vi "Reproductor.vi"() -> ()   [LabVIEW 2016]
uses:
  <vilib>/sound2/lvsound2.llb/Sound Data Format.ctl
  <vilib>/sound2/lvsound2.llb/Sound File Position.ctl
  <vilib>/sound2/lvsound2.llb/Sampling Mode.ctl
  <vilib>/Analysis/baseanly.llb/Mean (DBL).vi
  <vilib>/sound2/lvsound2.llb/Sound File Read Open.vi
  <vilib>/sound2/lvsound2.llb/Sound File Info (refnum).vi
  <vilib>/sound2/lvsound2.llb/Sound File Read (DBL).vi
  <vilib>/measure/matone.llb/Extract Single Tone Information N Chan.vi
  <vilib>/measure/maspectr.llb/FFT Spectrum (Mag-Phase) for N Chan.vi
  <vilib>/sound2/lvsound2.llb/Sound Output Write (DBL).vi
  <vilib>/measure/NI_MAPro.lvlib
  <vilib>/Analysis/NI_AALBase.lvlib
panel:
  in  "Skip Forward Button":bool
  in  "Seek Forward Button":bool
  in  "Pause Button":bool
  in  "Play Button":bool
  in  "Seek Back Button":bool
  in  "Skip Back Button":bool
  in  "posicion":dbl(slide) scale=0.0..10.0
  out "Color Box":u32(colorbox)
  out "Waveform Chart":cluster{"mean":dbl, "detected frequency":dbl}(graph)
  out "Waveform Graph 2":cluster{"f0":dbl, "df":dbl, "magnitude":dbl[]}[](graph)
  in  "stop":bool
  out "Waveform Graph":waveform(dbl)[](graph)
  out "sound format":T1={"sample rate (S/s)"=22050.0, "number of channels"=2, "bits per sample"=16}
  out "total number of samples/ch":u32
  in  "path":path=path "C:/Users/jesus/Desktop/Reproductor/Shawn Mendes  Bad Reputation    Traducido al Español.wav"
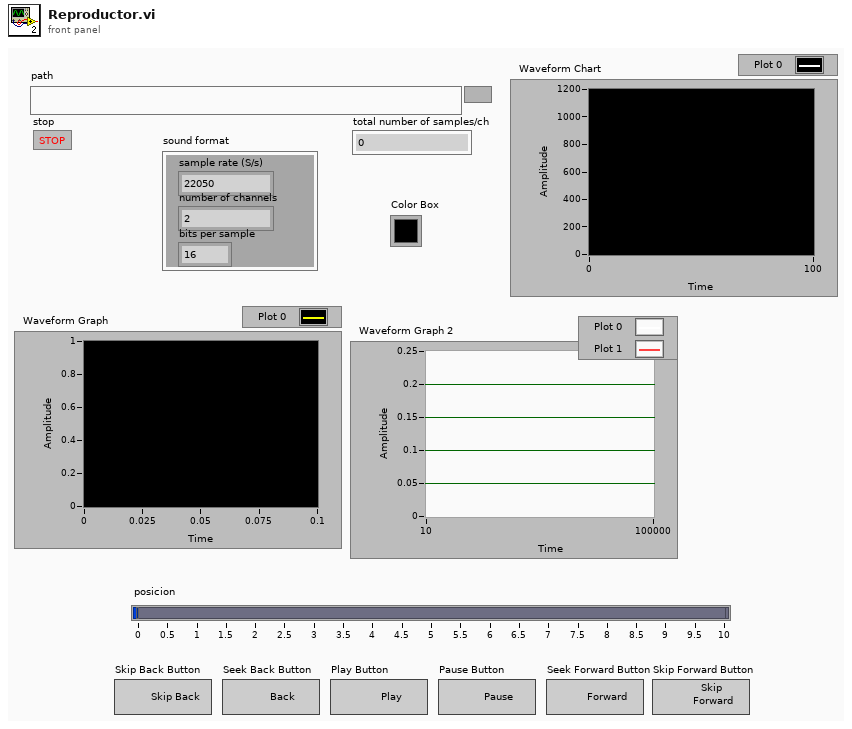
[diagram p1: front panel]
types:
  T1 = typedef "Sound Data Format.ctl" = cluster{"sample rate (S/s)":dbl, "number of channels":i32, "bits per sample":i32}
  T2 = typedef "Sampling Mode.ctl" = i32
  T3 = typedef "Sound File Position.ctl" = u16
  T4 = typedef "Sound File Refnum.ctl" = refnum<file>
  T5 = typedef "Sound Output Task ID.ctl" = u32
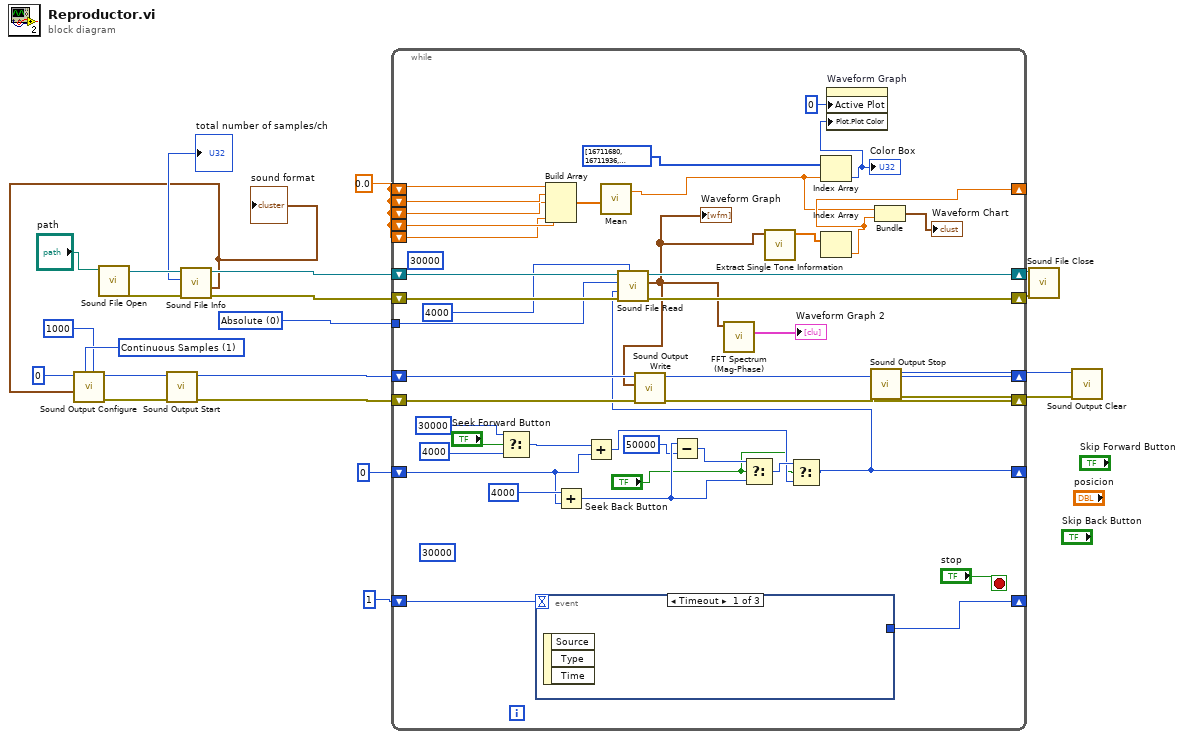
[diagram p0: block diagram]
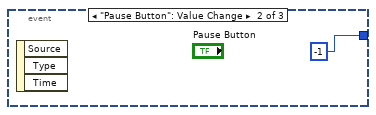
[diagram p2: hidden frame]
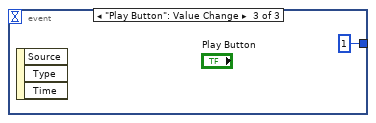
[diagram p3: hidden frame]
diagram:
  w3 = 0.0 ("detected frequency")
  w13 = T2 1 items=["Finite Samples", "Continuous Samples"] ("sample mode")
  w16 = T3 0 items=["Absolute"=0, "Relative"=2] ("position mode")
  n1 = call-poly <vilib>:"Sound File Open.vi"("path"="path") -> ("error out"=w22:errorcluster, "sound file refnum"=w23:T4)  [unwired: 9 in]
  n2 = call-poly <vilib>:"Sound File Info.vi"("error in (no error)"=w22, "sound file refnum"=w23) -> ("error out"=w19:errorcluster, "sound format"=w14:T1, "total number of samples/ch"=→"total number of samples/ch":u32, "sound file refnum out"=w20:T4)  [unwired: 6 in]
  "sound format" <- w14
  n3 = call <vilib>:"Sound Output Configure.vi"("number of samples/ch"=1000, "sample mode"=w13, "sound format"=w14, "device ID"=u32 0) -> ("error out"=w10:errorcluster, "task ID"=w11:T5)  [unwired: 6 in]
  n4 = call <vilib>:"Sound Output Start.vi"("error in (no error)"=w10, "task ID"=w11) -> ("error out"=w8:errorcluster, "task ID out"=w9:T5)  [unwired: 8 in]
  n5 = while {
    tunnel: w16 -> [w61]
    shift-right: [w63] -> w18
    shift-left: w20 -> [w65]
    shift-right: [w62] -> w17
    shift-left: w19 -> [w64]
    shift-right: [w58] -> w7
    shift-left: w9 -> [w60]
    shift-right: [w57] -> w5
    shift-left: w8 -> [w59]
    shift-right: [w46] -> _
    shift-left: w3 -> [w50]
    shift-left: w3 -> [w51]
    shift-left: w3 -> [w49]
    shift-left: w3 -> [w48]
    shift-left: w3 -> [w41]
    shift-right: [w27] -> _
    shift-left: 0 -> [w32]
    shift-right: [w40] -> _
    shift-left: 1 -> [w39]
    stop <- "stop" stop-if-true
    (unwired) 30000 ("number of samples/ch (-1: all)")
    (unwired) 30000 ("number of samples/ch (-1: all)")
    n6 = Select(t=30000 ("number of samples/ch (-1: all)"), s="Seek Forward Button", f=4000) -> (s? t:f=w38:i32)
    n7 = event shown="[0] Timeout" {
      selector: _ -> [_ _ _]
      dyn-events: _ -> [_ _ _]
      timeout: w39 -> [_ _ _]
      tunnel: [_ -1 1] -> w40
      event Timeout {
        n8 = event-data() -> ()  [unwired: 1 in, 3 out]
      }
      event "Pause Button": Value Change {
        n9 = event-data() -> ()  [unwired: 1 in, 3 out]
      }
      event "Play Button": Value Change {
        n10 = event-data() -> ()  [unwired: 1 in, 3 out]
      }
    }
    n11 = Build Array(w50, w51, w49, w48, w41) -> (w47:dbl[])
    n12 = Add(x=4000, y=w32) -> (x+y=w30:i32)
    n13 = Add(x=w38, y=w32) -> (x+y=w26:i32)
    n14 = call-poly <vilib>:"Mean.vi"("X"=w47) -> ("mean"=w45:dbl)  [unwired: 1 out]
    n15 = Subtract(x=w30, y=50000 ("x")) -> (x-y=w31:i32)
    n16 = Select(t=w31, s="Seek Back Button", f=w30) -> (s? t:f=w28:i32)
    n17 = Select(t=w28, s="Seek Back Button", f=w26) -> (s? t:f=w27:i32)
    n18 = call-poly <vilib>:"Sound File Read.vi"("number of samples/ch (-1: all)"=4000, "error in (no error)"=w64, "position offset"=w27, "position mode"=w61, "sound file refnum"=w65) -> ("error out"=w62:errorcluster, "data"=w54:waveform(dbl)[], "sound file refnum out"=w63:T4)  [unwired: 2 in, 2 out]
    "Waveform Graph" <- w54
    n19 = call-poly <vilib>:"Sound Output Write.vi"("error in (no error)"=w59, "data"=w54, "task ID"=w60) -> ("error out"=w57:errorcluster, "task ID out"=w58:T5)  [unwired: 7 in]
    n20 = call-poly <vilib>:"FFT Spectrum (Mag-Phase).vi"("time signals"=w54) -> ("magnitudes"=→"Waveform Graph 2":cluster{"f0":dbl, "df":dbl, "magnitude":dbl[]}[])  [unwired: 6 in, 4 out]
    n21 = call-poly <vilib>:"Extract Single Tone Information.vi"("time signals in"=w54) -> ("detected frequencies"=w53:dbl[])  [unwired: 5 in, 5 out]
    n22 = Index Array(array=u32[] [16711680, 16711936, 16712192, 16712448, 16712704, 16712960, 16713216, 16713472, 16713728, 16713984, 16714240, 16714496, 16714752, 16715008, 16715264, 16715520, 16715776, 16716032, 16716288, 16716544, 16716800, 16717056, 16717312, 16717568, 16717824, 16718080, 16718336, 16718592, 16718848, 16719104, 16719360, 16719616, 16719872, 16720128, 16720384, 16720640, 16720896, 16721152, 16721408, 16721664, 16721920, 16722176, 16722432, 16722688, 16722944, 16723200, 16723456, 16723712, 16723968, 16724224, 16724480, 16724736, 16724992, 16725248, 16725504, 16725760, 16726016, 16726272, 16726528, 16726784, 16727040, 16727296, 16727552, 16727808, 16728064, 16728320, 16728576, 16728832, 16729088, 16729344, 16729600, 16729856, 16730112, 16730368, 16730624, 16730880, 16731136, 16731392, 16731648, 16731904, 16732160, 16732416, 16732672, 16732928, 16733184, 16733440, 16733696, 16733952, 16734208, 16734464, 16734720, 16734976, 16735232, 16735488, 16735744, 16736000, 16736256, 16736512, 16736768, 16737024, 16737280, 16737536, 16737792, 16738048, 16738304, 16738560, 16738816, 16739072, 16739328, 16739584, 16739840, 16740096, 16740352, 16740608, 16740864, 16741120, 16741376, 16741632, 16741888, 16742144, 16742400, 16742656, 16742912, 16743168, 16743424, 16743680, 16743936, 16744192, 16744448, 16744704, 16744960, 16745216, 16745472, 16745728, 16745984, 16746240, 16746496, 16746752, 16747008, 16747264, 16747520, 16747776, 16748032, 16748288, 16748544, 16748800, 16749056, 16749312, 16749568, 16749824, 16750080, 16750336, 16750592, 16750848, 16751104, 16751360, 16751616, 16751872, 16752128, 16752384, 16752640, 16752896, 16753152, 16753408, 16753664, 16753920, 16754176, 16754432, 16754688, 16754944, 16755200, 16755456, 16755712, 16755968, 16756224, 16756480, 16756736, 16756992, 16757248, 16757504, 16757760, 16758016, 16758272, 16758528, 16758784, 16759040, 16759296, 16759552, 16759808, 16760064, 16760320, 16760576, 16760832, 16761088, 16761344, 16761600, 16761856, 16762112, 16762368, 16762624, 16762880, 16763136, 16763392, 16763648, 16763904, 16764160, 16764416, 16764672, 16764928, 16765184, 16765440, 16765696, 16765952, 16766208, 16766464, 16766720, 16766976, 16767232, 16767488, 16767744, 16768000, 16768256, 16768512, 16768768, 16769024, 16769280, 16769536, 16769792, 16770048, 16770304, 16770560, 16770816, 16771072, 16771328, 16771584, 16771840, 16772096, 16772352, 16772608, 16772864, 16773120, 16773376, 16773632, 16773888, 16774144, 16774400, 16774656, 16774912, 16775168, 16775424, 16775680, 16775936, 16776192, 16776448, 16776704, 16776960, 16711424, 16645888, 16580352, 16514816, 16449280, 16383744, 16318208, 16252672, 16187136, 16121600, 16056064, 15990528, 15924992, 15859456, 15793920, 15728384, 15662848, 15597312, 15531776, 15466240, 15400704, 15335168, 15269632, 15204096, 15138560, 15073024, 15007488, 14941952, 14876416, 14810880, 14745344, 14679808, 14614272, 14548736, 14483200, 14417664, 14352128, 14286592, 14221056, 14155520, 14089984, 14024448, 13958912, 13893376, 13827840, 13762304, 13696768, 13631232, 13565696, 13500160, 13434624, 13369088, 13303552, 13238016, 13172480, 13106944, 13041408, 12975872, 12910336, 12844800, 12779264, 12713728, 12648192, 12582656, 12517120, 12451584, 12386048, 12320512, 12254976, 12189440, 12123904, 12058368, 11992832, 11927296, 11861760, 11796224, 11730688, 11665152, 11599616, 11534080, 11468544, 11403008, 11337472, 11271936, 11206400, 11140864, 11075328, 11009792, 10944256, 10878720, 10813184, 10747648, 10682112, 10616576, 10551040, 10485504, 10419968, 10354432, 10288896, 10223360, 10157824, 10092288, 10026752, 9961216, 9895680, 9830144, 9764608, 9699072, 9633536, 9568000, 9502464, 9436928, 9371392, 9305856, 9240320, 9174784, 9109248, 9043712, 8978176, 8912640, 8847104, 8781568, 8716032, 8650496, 8584960, 8519424, 8453888, 8388352, 8322816, 8257280, 8191744, 8126208, 8060672, 7995136, 7929600, 7864064, 7798528, 7732992, 7667456, 7601920, 7536384, 7470848, 7405312, 7339776, 7274240, 7208704, 7143168, 7077632, 7012096, 6946560, 6881024, 6815488, 6749952, 6684416, 6618880, 6553344, 6487808, 6422272, 6356736, 6291200, 6225664, 6160128, 6094592, 6029056, 5963520, 5897984, 5832448, 5766912, 5701376, 5635840, 5570304, 5504768, 5439232, 5373696, 5308160, 5242624, 5177088, 5111552, 5046016, 4980480, 4914944, 4849408, 4783872, 4718336, 4652800, 4587264, 4521728, 4456192, 4390656, 4325120, 4259584, 4194048, 4128512, 4062976, 3997440, 3931904, 3866368, 3800832, 3735296, 3669760, 3604224, 3538688, 3473152, 3407616, 3342080, 3276544, 3211008, 3145472, 3079936, 3014400, 2948864, 2883328, 2817792, 2752256, 2686720, 2621184, 2555648, 2490112, 2424576, 2359040, 2293504, 2227968, 2162432, 2096896, 2031360, 1965824, 1900288, 1834752, 1769216, 1703680, 1638144, 1572608, 1507072, 1441536, 1376000, 1310464, 1244928, 1179392, 1113856, 1048320, 982784, 917248, 851712, 786176, 720640, 655104, 589568, 524032, 458496, 392960, 327424, 261888, 196352, 130816, 65280, 65281, 65282, 65283, 65284, 65285, 65286, 65287, 65288, 65289, 65290, 65291, 65292, 65293, 65294, 65295, 65296, 65297, 65298, 65299, 65300, 65301, 65302, 65303, 65304, 65305, 65306, 65307, 65308, 65309, 65310, 65311, 65312, 65313, 65314, 65315, 65316, 65317, 65318, 65319, 65320, 65321, 65322, 65323, 65324, 65325, 65326, 65327, 65328, 65329, 65330, 65331, 65332, 65333, 65334, 65335, 65336, 65337, 65338, 65339, 65340, 65341, 65342, 65343, 65344, 65345, 65346, 65347, 65348, 65349, 65350, 65351, 65352, 65353, 65354, 65355, 65356, 65357, 65358, 65359, 65360, 65361, 65362, 65363, 65364, 65365, 65366, 65367, 65368, 65369, 65370, 65371, 65372, 65373, 65374, 65375, 65376, 65377, 65378, 65379, 65380, 65381, 65382, 65383, 65384, 65385, 65386, 65387, 65388, 65389, 65390, 65391, 65392, 65393, 65394, 65395, 65396, 65397, 65398, 65399, 65400, 65401, 65402, 65403, 65404, 65405, 65406, 65407, 65408, 65409, 65410, 65411, 65412, 65413, 65414, 65415, 65416, 65417, 65418, 65419, 65420, 65421, 65422, 65423, 65424, 65425, 65426, 65427, 65428, 65429, 65430, 65431, 65432, 65433, 65434, 65435, 65436, 65437, 65438, 65439, 65440, 65441, 65442, 65443, 65444, 65445, 65446, 65447, 65448, 65449, 65450, 65451, 65452, 65453, 65454, 65455, 65456, 65457, 65458, 65459, 65460, 65461, 65462, 65463, 65464, 65465, 65466, 65467, 65468, 65469, 65470, 65471, 65472, 65473, 65474, 65475, 65476, 65477, 65478, 65479, 65480, 65481, 65482, 65483, 65484, 65485, 65486, 65487, 65488, 65489, 65490, 65491, 65492, 65493, 65494, 65495, 65496, 65497, 65498, 65499, 65500, 65501, 65502, 65503, 65504, 65505, 65506, 65507, 65508, 65509, 65510, 65511, 65512, 65513, 65514, 65515, 65516, 65517, 65518, 65519, 65520, 65521, 65522, 65523, 65524, 65525, 65526, 65527, 65528, 65529, 65530, 65531, 65532, 65533, 65534, 65535, 65279, 65023, 64767, 64511, 64255, 63999, 63743, 63487, 63231, 62975, 62719, 62463, 62207, 61951, 61695, 61439, 61183, 60927, 60671, 60415, 60159, 59903, 59647, 59391, 59135, 58879, 58623, 58367, 58111, 57855, 57599, 57343, 57087, 56831, 56575, 56319, 56063, 55807, 55551, 55295, 55039, 54783, 54527, 54271, 54015, 53759, 53503, 53247, 52991, 52735, 52479, 52223, 51967, 51711, 51455, 51199, 50943, 50687, 50431, 50175, 49919, 49663, 49407, 49151, 48895, 48639, 48383, 48127, 47871, 47615, 47359, 47103, 46847, 46591, 46335, 46079, 45823, 45567, 45311, 45055, 44799, 44543, 44287, 44031, 43775, 43519, 43263, 43007, 42751, 42495, 42239, 41983, 41727, 41471, 41215, 40959, 40703, 40447, 40191, 39935, 39679, 39423, 39167, 38911, 38655, 38399, 38143, 37887, 37631, 37375, 37119, 36863, 36607, 36351, 36095, 35839, 35583, 35327, 35071, 34815, 34559, 34303, 34047, 33791, 33535, 33279, 33023, 32767, 32511, 32255, 31999, 31743, 31487, 31231, 30975, 30719, 30463, 30207, 29951, 29695, 29439, 29183, 28927, 28671, 28415, 28159, 27903, 27647, 27391, 27135, 26879, 26623, 26367, 26111, 25855, 25599, 25343, 25087, 24831, 24575, 24319, 24063, 23807, 23551, 23295, 23039, 22783, 22527, 22271, 22015, 21759, 21503, 21247, 20991, 20735, 20479, 20223, 19967, 19711, 19455, 19199, 18943, 18687, 18431, 18175, 17919, 17663, 17407, 17151, 16895, 16639, 16383, 16127, 15871, 15615, 15359, 15103, 14847, 14591, 14335, 14079, 13823, 13567, 13311, 13055, 12799, 12543, 12287, 12031, 11775, 11519, 11263, 11007, 10751, 10495, 10239, 9983, 9727, 9471, 9215, 8959, 8703, 8447, 8191, 7935, 7679, 7423, 7167, 6911, 6655, 6399, 6143, 5887, 5631, 5375, 5119, 4863, 4607, 4351, 4095, 3839, 3583, 3327, 3071, 2815, 2559, 2303, 2047, 1791, 1535, 1279, 1023, 767, 511, 255, 65791, 131327, 196863, 262399, 327935, 393471, 459007, 524543, 590079, 655615, 721151, 786687, 852223, 917759, 983295, 1048831, 1114367, 1179903, 1245439, 1310975, 1376511, 1442047, 1507583, 1573119, 1638655, 1704191, 1769727, 1835263, 1900799, 1966335, 2031871, 2097407, 2162943, 2228479, 2294015, 2359551, 2425087, 2490623, 2556159, 2621695, 2687231, 2752767, 2818303, 2883839, 2949375, 3014911, 3080447, 3145983, 3211519, 3277055, 3342591, 3408127, 3473663, 3539199, 3604735, 3670271, 3735807, 3801343, 3866879, 3932415, 3997951, 4063487, 4129023, 4194559, 4260095, 4325631, 4391167, 4456703, 4522239, 4587775, 4653311, 4718847, 4784383, 4849919, 4915455, 4980991, 5046527, 5112063, 5177599, 5243135, 5308671, 5374207, 5439743, 5505279, 5570815, 5636351, 5701887, 5767423, 5832959, 5898495, 5964031, 6029567, 6095103, 6160639, 6226175, 6291711, 6357247, 6422783, 6488319, 6553855, 6619391, 6684927, 6750463, 6815999, 6881535, 6947071, 7012607, 7078143, 7143679, 7209215, 7274751, 7340287, 7405823, 7471359, 7536895, 7602431, 7667967, 7733503, 7799039, 7864575, 7930111, 7995647, 8061183, 8126719, 8192255, 8257791, 8323327, 8388863, 8454399, 8519935, 8585471, 8651007, 8716543, 8782079, 8847615, 8913151, 8978687, 9044223, 9109759, 9175295, 9240831, 9306367, 9371903, 9437439, 9502975, 9568511, 9634047, 9699583, 9765119, 9830655, 9896191, 9961727, 10027263, 10092799, 10158335, 10223871, 10289407, 10354943, 10420479, 10486015, 10551551, 10617087, 10682623, 10748159, 10813695, 10879231, 10944767, 11010303, 11075839, 11141375, 11206911, 11272447, 11337983, 11403519, 11469055, 11534591, 11600127, 11665663, 11731199, 11796735, 11862271, 11927807, 11993343, 12058879, 12124415, 12189951, 12255487, 12321023, 12386559, 12452095, 12517631, 12583167, 12648703, 12714239, 12779775, 12845311, 12910847, 12976383, 13041919, 13107455, 13172991, 13238527, 13304063, 13369599, 13435135, 13500671, 13566207, 13631743, 13697279, 13762815, 13828351, 13893887, 13959423, 14024959, 14090495, 14156031, 14221567, 14287103, 14352639, 14418175, 14483711, 14549247, 14614783, 14680319, 14745855, 14811391, 14876927, 14942463, 15007999, 15073535, 15139071, 15204607, 15270143, 15335679, 15401215, 15466751, 15532287, 15597823, 15663359, 15728895, 15794431, 15859967, 15925503, 15991039, 16056575, 16122111, 16187647, 16253183, 16318719, 16384255, 16449791, 16515327, 16580863, 16646399, 16711935, 16711934, 16711933, 16711932, 16711931, 16711930, 16711929, 16711928, 16711927, 16711926, 16711925, 16711924, 16711923, 16711922, 16711921, 16711920, 16711919, 16711918, 16711917, 16711916, 16711915, 16711914, 16711913, 16711912, 16711911, 16711910, 16711909, 16711908, 16711907, 16711906, 16711905, 16711904, 16711903, 16711902, 16711901, 16711900, 16711899, 16711898, 16711897, 16711896, 16711895, 16711894, 16711893, 16711892, 16711891, 16711890, 16711889, 16711888, 16711887, 16711886, 16711885, 16711884, 16711883, 16711882, 16711881, 16711880, 16711879, 16711878, 16711877, 16711876, 16711875, 16711874, 16711873, 16711872, 16711871, 16711870, 16711869, 16711868, 16711867, 16711866, 16711865, 16711864, 16711863, 16711862, 16711861, 16711860, 16711859, 16711858, 16711857, 16711856, 16711855, 16711854, 16711853, 16711852, 16711851, 16711850, 16711849, 16711848, 16711847, 16711846, 16711845, 16711844, 16711843, 16711842, 16711841, 16711840, 16711839, 16711838, 16711837, 16711836, 16711835, 16711834, 16711833, 16711832, 16711831, 16711830, 16711829, 16711828, 16711827, 16711826, 16711825, 16711824, 16711823, 16711822, 16711821, 16711820, 16711819, 16711818, 16711817, 16711816, 16711815, 16711814, 16711813, 16711812, 16711811, 16711810, 16711809, 16711808, 16711807, 16711806, 16711805, 16711804, 16711803, 16711802, 16711801, 16711800, 16711799, 16711798, 16711797, 16711796, 16711795, 16711794, 16711793, 16711792, 16711791, 16711790, 16711789, 16711788, 16711787, 16711786, 16711785, 16711784, 16711783, 16711782, 16711781, 16711780, 16711779, 16711778, 16711777, 16711776, 16711775, 16711774, 16711773, 16711772, 16711771, 16711770, 16711769, 16711768, 16711767, 16711766, 16711765, 16711764, 16711763, 16711762, 16711761, 16711760, 16711759, 16711758, 16711757, 16711756, 16711755, 16711754, 16711753, 16711752, 16711751, 16711750, 16711749, 16711748, 16711747, 16711746, 16711745, 16711744, 16711743, 16711742, 16711741, 16711740, 16711739, 16711738, 16711737, 16711736, 16711735, 16711734, 16711733, 16711732, 16711731, 16711730, 16711729, 16711728, 16711727, 16711726, 16711725, 16711724, 16711723, 16711722, 16711721, 16711720, 16711719, 16711718, 16711717, 16711716, 16711715, 16711714, 16711713, 16711712, 16711711, 16711710, 16711709, 16711708, 16711707, 16711706, 16711705, 16711704, 16711703, 16711702, 16711701, 16711700, 16711699, 16711698, 16711697, 16711696, 16711695, 16711694, 16711693, 16711692, 16711691, 16711690, 16711689, 16711688, 16711687, 16711686, 16711685, 16711684, 16711683, 16711682, 16711681] ("Array 2"), index=w45) -> (element=w43:u32)
    "Color Box" <- w43
    n23 = Index Array(array=w53) -> (element=w46:dbl)  [unwired: 1 in]
    n24 = property on="Waveform Graph" class="WFGraph (strict)"("Active Plot"=u32 0, "Plot.Plot Color"=w43) -> ()  [unwired: 2 in, 2 out]
    n25 = Bundle("mean"=w45, "detected frequency"=w46) -> (→"Waveform Chart":cluster{"mean":dbl, "detected frequency":dbl})  [unwired: 1 in]
  }
  n26 = call <vilib>:"Sound Output Stop.vi"("error in (no error)"=w5, "task ID"=w7) -> ("error out"=w4:errorcluster, "task ID out"=w6:T5)  [unwired: 8 in]
  n27 = call <vilib>:"Sound File Close.vi"("error in (no error)"=w17, "sound file refnum"=w18) -> ()  [unwired: 9 in, 1 out]
  n28 = call <vilib>:"Sound Output Clear.vi"("error in (no error)"=w4, "task ID"=w6) -> ()  [unwired: 9 in, 1 out]
